vi "detectFluidTouch.vi"(5 "which manipulator":T1(ring), 6 "lowest position":i32[](array[numeric]), 7 "avg peak height Refnum":refnum<vi>, 8 "error in":errorcluster, 9 "mclamp cluster":T2, 10 "Multiclamp Handle in":u32=722860, 11 "manip in":T3={"Actuator COM"="COM14", "Actuator type"=enum."Scientifica"}) -> (0 "error out":errorcluster, 2 "detected":bool, 3 "manip out":T3={"Actuator COM"="COM14", "Actuator type"=enum."Scientifica"})   [LabVIEW 2015]
uses:
  controls/scientifica_commands.ctl
  multiBot/patcherBot/AxMultiClampMsg.dll
  controls/actuator_type.ctl
  controls/actuator_cluster.ctl
panel:
  in  "speed":string="-5000"
  out "Z pos (steps)":i32
  in  "stop":bool
  out "Waveform\nChart":dbl(graph)
  # "changed from -10000 (7-9-17)\nfor dual patching"
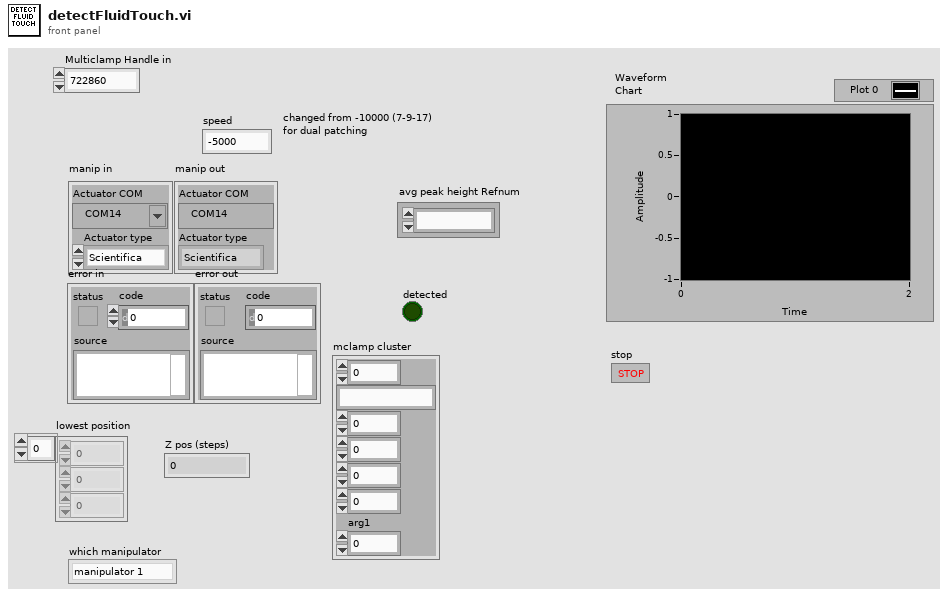
[diagram p1: front panel]
types:
  T1 = enum16{"manipulator 1", "manipulator 2", "manipulator 3", "manipulator 4"}
  T2 = cluster{u32, string, i32, u32, u32, u32, "arg1":i32}
  T3 = typedef "actuator_cluster.ctl" = cluster{"Actuator COM":refnum<visa-resource-name>, "Actuator type":T4}
  T4 = typedef "actuator_type.ctl" = enum16{"Scientifica", "Sutter", "Demo", "Off"}
  T5 = typedef "scientifica_commands.ctl" = enum16{"ANGLE", "INSET", "FIRST", "ZERO", "Pz", "P", "absz", "ACC", "TOP", "STOP", "rel", "relz", "abs", "IN", "vj", "APROACH", "OBJS", "OBJU", "OUT", "OBJ", "OBJL", "SET", "OBJD", "STEP", "SETSTEP", "S", "UUX", "UUY", "UUZ"}
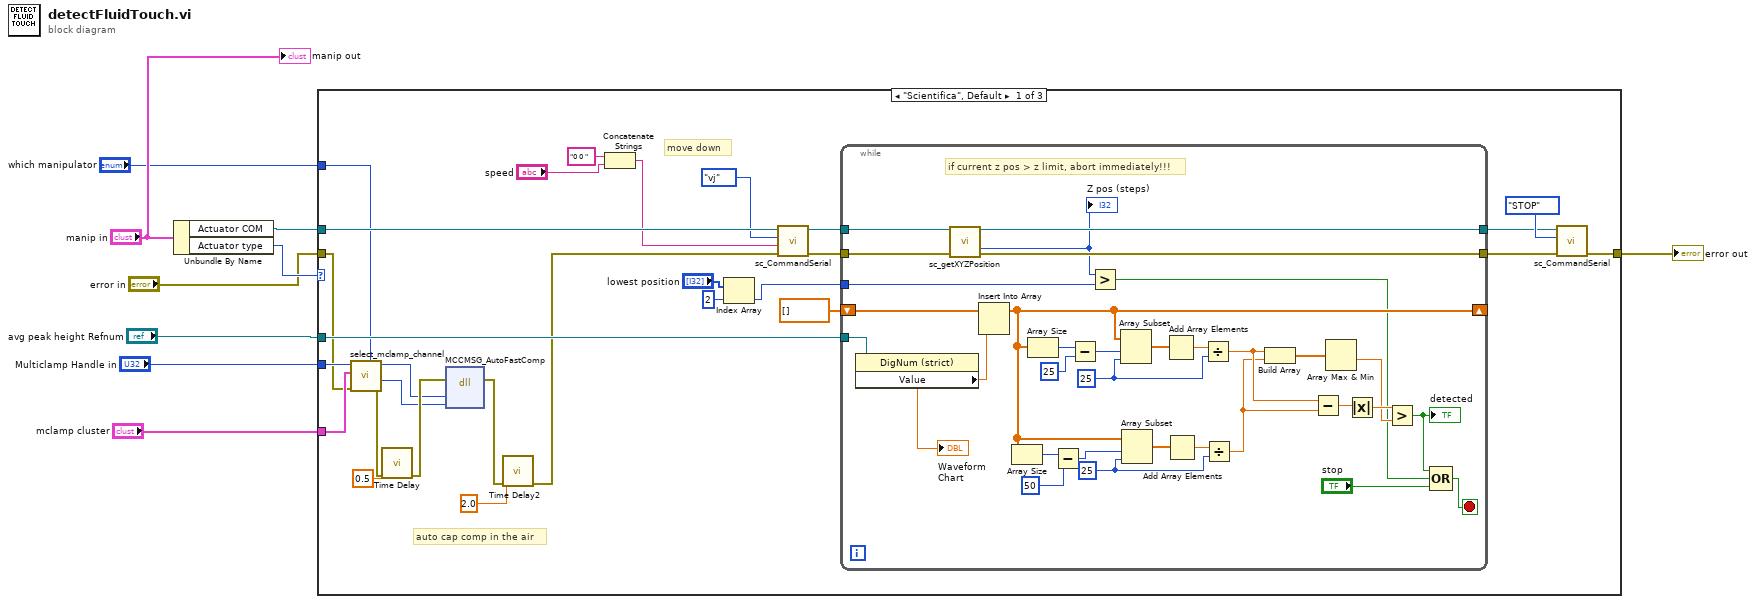
[diagram p0: block diagram]
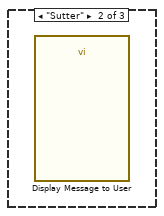
[diagram p2: hidden frame]
diagram:
  n1 = Unbundle By Name("manip in") -> ("Actuator COM"=w9:refnum<visa-resource-name>, "Actuator type"=w8:T4)
  n2 = case shown="\"Scientifica\", Default" w8 {
    tunnel: w9 -> [w37 _ _]
    tunnel: "error in" -> [w10 _ _]
    tunnel: "avg peak height Refnum" -> [w30 _ _]
    tunnel: [w29 _ _] -> w4
    tunnel: "Multiclamp Handle in" -> [w15 _ _]
    tunnel: "mclamp cluster" -> [w14 _ _]
    tunnel: "which manipulator" -> [w12 _ _]
    frame "Scientifica", Default {
      # "auto cap comp in the air"
      # "move down"
      n3 = call "select_mclamp_channel.vi"("which manipulator"=w12, "error in (no error)"=w10, "mclamp cluster"=w14, "Multiclamp Handle In"=w15) -> ("error out"=w11:errorcluster, "error"=w13:i32, "Multiclamp Handle out"=w16:u32)  [unwired: 5 in]
      n4 = call "Time Delay"("error in (no error)"=w11, "Delay Time (s)"=0.5) -> ("error out"=w22:errorcluster)  [unwired: 9 in]
      n5 = dll-call lib="C:/multiBot/patcherBot/AxMultiClampMsg.dll" fn="MCCMSG_AutoFastComp"(error in=w22, "handle"=w16, "error"=w13) -> (error out=w21:errorcluster)  [unwired: 5 in, 1 out]
      n6 = call "Time Delay2"("error in (no error)"=w21, "Delay Time (s)"=2.0) -> ("error out"=w20:errorcluster)  [unwired: 9 in]
      n7 = Concatenate Strings("0 0 " ("string"), "speed") -> (w17:string)
      n8 = Index Array(array="lowest position", index=2) -> (element=w26:i32)
      n9 = call "sc_CommandSerial.vi"("error in (no error)"=w20, "argument"=w17, "Scientifica commands"=scientifica_commands."vj", "VISA handle"=w37) -> ("error out"=w32:errorcluster, "Dup. VISA handle"=w34:refnum<visa-resource-name>)  [unwired: 4 in, 2 out]
      n10 = while {
        shift-right: [w43] -> _
        shift-left: dbl[] [] -> [w69]
        tunnel: w34 -> [w50]
        tunnel: [w48] -> w33
        tunnel: w32 -> [w49]
        tunnel: [w47] -> w31
        tunnel: w30 -> [w45]
        tunnel: w26 -> [w39]
        stop <- w51 stop-if-true
        w65 = 25 ("length")
        w66 = 25 ("length")
        # "if current z pos > z limit, abort immediately!!!"
        n11 = property class="DigNum (strict)"(reference=w45) -> ("Value"=w44:dbl)  [unwired: 1 in, 2 out]
        "Waveform\nChart" <- w44
        n12 = call "sc_getXYZPosition.vi"("VISA handle 2"=w50, "error in (no error) 2"=w49) -> ("Dup. VISA handle 2"=w48:refnum<visa-resource-name>, "Z pos (steps)"=w46:i32, "error out 2"=w47:errorcluster)  [unwired: 9 in, 2 out]
        "Z pos (steps)" <- w46
        n13 = Insert Into Array(array=w69, new element=w44) -> (w43:dbl[])  [unwired: 1 in]
        n14 = Array Size(array=w43) -> (size(s)=w42:i32)
        n15 = Array Size(array=w43) -> (size(s)=w62:i32)
        n16 = Subtract(x=w42, y=50) -> (x-y=w40:i32)
        n17 = Subtract(x=w62, y=25) -> (x-y=w60:i32)
        n18 = Greater?(x=w46, y=w39) -> (0:w38:bool)
        n19 = Array Subset(array=w43, index=w60, length=w66) -> (w68:dbl[])
        n20 = Array Subset(array=w43, index=w40, length=w65) -> (w63:dbl[])
        n21 = Add Array Elements(numeric array=w68) -> (sum=w67:dbl)
        n22 = Add Array Elements(numeric array=w63) -> (sum=w64:dbl)
        n23 = Divide(x=w67, y=w66) -> (x/y=w57:dbl)
        n24 = Divide(x=w64, y=w65) -> (x/y=w56:dbl)
        n25 = Build Array(w57, w56) -> (w55:dbl[])
        n26 = Subtract(x=w57, y=w56) -> (x-y=w59:dbl)
        n27 = Array Max & Min(array=w55) -> (min value=w54:dbl)  [unwired: 3 out]
        n28 = Absolute Value(x=w59) -> (abs(x)=w58:dbl)
        n29 = Greater?(x=w58, y=w54) -> (0:w52:bool)
        "detected" <- w52
        n30 = Compound Arithmetic op=OR(w52, w38, "stop") -> (w51:bool)
      }
      n31 = call "sc_CommandSerial.vi"("error in (no error)"=w31, "Scientifica commands"=scientifica_commands."STOP", "VISA handle"=w33) -> ("error out"=w29:errorcluster)  [unwired: 5 in, 3 out]
    }
    frame "Sutter" {
      n32 = call "Display Message to User"() -> ()  [unwired: 10 in, 2 out]
    }
    frame "Demo" {
    }
  }
  "error out" <- w4
  "manip out" <- "manip in"
